vi "Read coninfo.vi"(8 "error in (no error)":errorcluster, 11 "SP in":refnum<class "Save messages PGserver.lvclass">) -> (0 "error out":errorcluster, 2 "conninfo":T1, 3 "SP out":refnum<class "Save messages PGserver.lvclass">)   [LabVIEW 2019, in "Save messages PGserver.lvclass"]
uses:
  Save messages PGserver.lvclass
  ctl/Coninfo.ctl
  Save messages PGserver.lvclass/Save messages PGserver.ctl
  PostgreSQL.lvlib
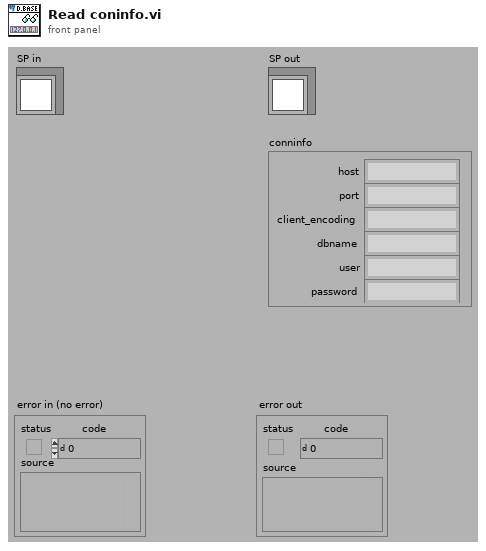
[diagram p1: front panel]
types:
  T1 = typedef "PostgreSQL.lvlib/Coninfo.ctl" = cluster{"host":string, "port":string, "client_encoding":string, "dbname":string, "user":string, "password":string}
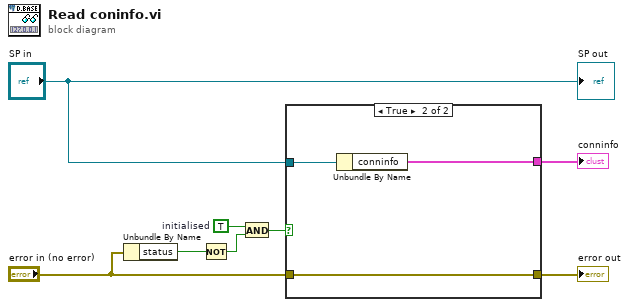
[diagram p0: block diagram]
diagram:
  w3 = TRUE  # initialised
  n1 = Unbundle By Name("error in (no error)") -> ("status"=w6:bool)
  n2 = Not(x=w6) -> (.not. x?=w5:bool)
  n3 = And(x=w3, y=w5) -> (x .and. y?=w7:bool)
  n4 = case shown="True" w7 {
    tunnel: [w9 w11] -> w8
    tunnel: "SP in" -> [_ w12]
    tunnel: "error in (no error)" -> [w9 w11]
    tunnel: [_ w10] -> w1
    frame False {
    }
    frame True {
      n5 = Unbundle By Name(w12) -> ("conninfo"=w10:T1)
    }
  }
  "error out" <- w8
  "conninfo" <- w1
  "SP out" <- "SP in"
